vi "DPOAEs_Cecilia_Casarini.vi"() -> ()   [LabVIEW 2015]
uses:
  <vilib>/Utility/error.llb/DialogType.ctl
  <vilib>/DAQmx/write.llb/DAQmx Write (Analog 1D Wfm NChan NSamp).vi
  <vilib>/DAQmx/read.llb/DAQmx Read (Analog Wfm 1Chan NSamp).vi
  <vilib>/addons/_NISVFA/_Baseband FFT/SVPO Power Spectrum (1 Ch DBL Array).vi
  <vilib>/addons/_NISVFA/_Baseband FFT/subVIs/svfa_Convert to One-Sided Power Spectrum.vi
  <vilib>/Analysis/2dsp.llb/Power Spectrum.vi
  <vilib>/Analysis/2dsp.llb/Power Spectrum (DBL).vi
  <vilib>/addons/_NISVFA/_Shared subVIs/Windowing/svfa_Scaled Time Domain Window (Array).vi
  <vilib>/Analysis/4window.llb/Force Window.vi
  <vilib>/Analysis/4window.llb/Force Window (DBL).vi
  <vilib>/Analysis/4window.llb/Exponential Window.vi
  <vilib>/Analysis/4window.llb/Exponential Window (DBL).vi
  <vilib>/DAQmx/create/channels.llb/DAQmx Create Channel (AI-Voltage-Basic).vi
  <vilib>/DAQmx/create/channels.llb/DAQmx Create Channel (AO-Voltage-Basic).vi
  <vilib>/DAQmx/configure/timing.llb/DAQmx Timing (Sample Clock).vi
  <vilib>/DAQmx/configure/trigger.llb/DAQmx Start Trigger (Digital Edge).vi
  <vilib>/DAQmx/miscellaneous.llb/DAQmx Fill In Error Info.vi
  <vilib>/addons/_NISVFA/_Spectrum Processing/subVIs/svfa_Spectrum Info Window to windowTd Type Def.vi
  <vilib>/Analysis/0measdsp.llb/Scaled Time Domain Window.vi
  <vilib>/Analysis/0measdsp.llb/Scaled Time Domain Window (DBL).vi
  <vilib>/Utility/error.llb/Error Cluster From Error Code.vi
panel:
  in  "Frequency of Sine Tone AO-1":dbl=1000.0 format="%0.2p"
  in  "Amplitude of Sine Tone AO-1":dbl=1.0 format="%0.2p"
  out "Non-aligned output/input waveforms":waveform(dbl)(graph)
  in  "Number of extra samples \nto READ from ADC":i32=200
  out "Input spectrum":cluster{"f0":dbl, "df":dbl, "magnitude":dbl[]}(graph)
  out "number of samples \nwritten per channel":u32
  in  "Frequency of Sine Tone AO-0 2":dbl=1000.0 format="%0.2p"
  in  "Amplitude of Sine Tone AO-0":dbl=1.0 format="%0.2p"
  in  "sampling info":cluster{"Fs":dbl, "samples in waveform":dbl}={"Fs"=204800.0, "samples in waveform"=1024.0} {"Fs" format="%.2p"}
  out "buffer size":i32
  in  "minimum value":dbl=-5.0 caption="Output Minimum Value" format="%0.2f"
  in  "maximum value":dbl=5.0 caption="Output Maximum Value" format="%0.2f"
  in  "physical channels":tag="PXI1Slot5/ao0" caption="Output Physical Channels"
  in  "Maximum Value":dbl=5.0 caption="Input Maximum Value" format="%0.2f"
  in  "Minimum Value":dbl=-5.0 caption="Input Minimum Value" format="%0.2f"
  in  "Physical Channel":tag="PXI1Slot5/ai0" caption="Input Physical Channel"
  out "Output waveform (samples)":waveform(dbl)[](graph)
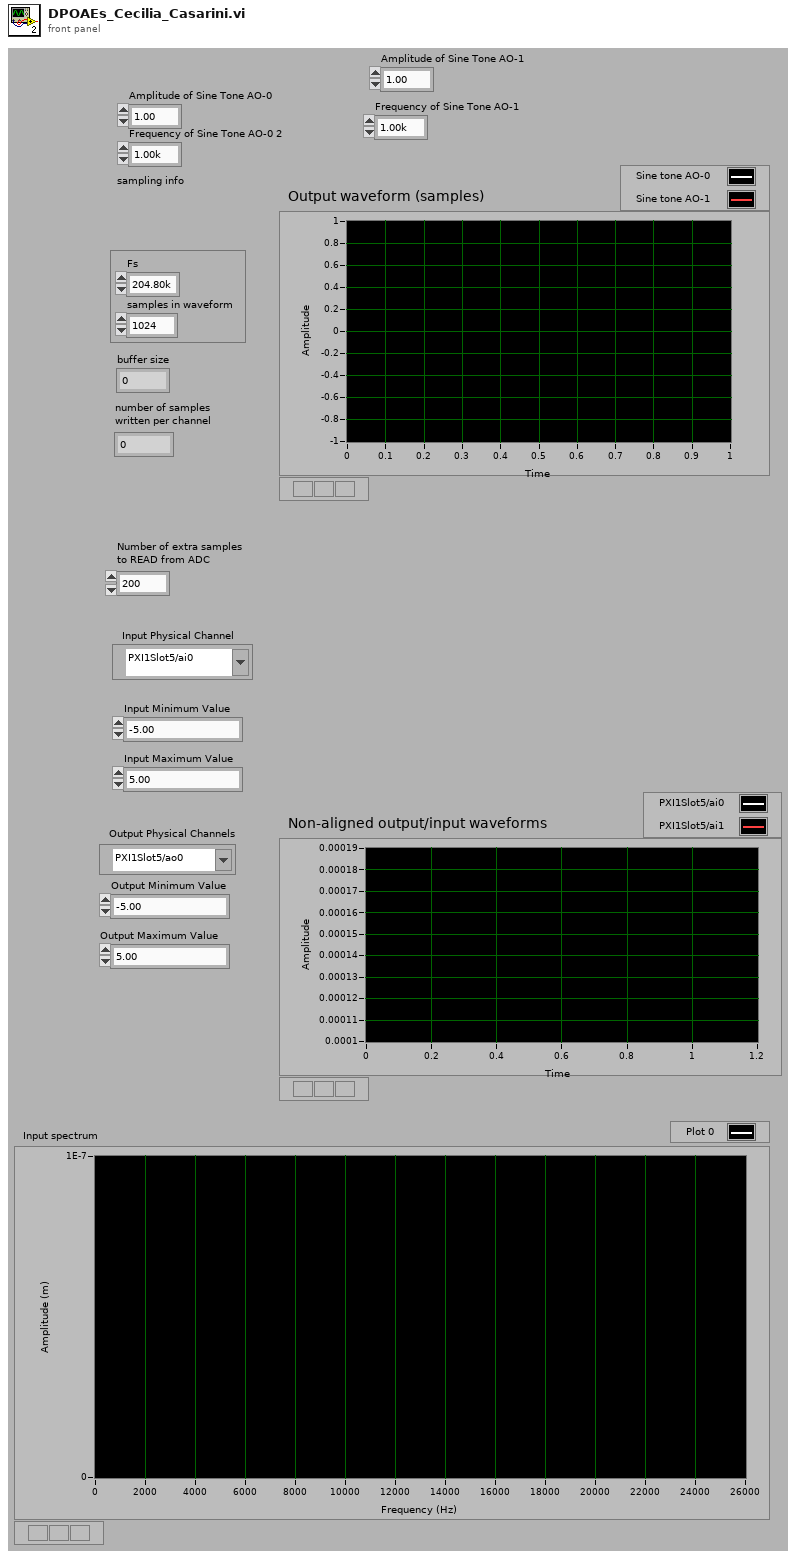
[diagram p1: front panel]
types:
  T1 = typedef "DialogType.ctl" = u16
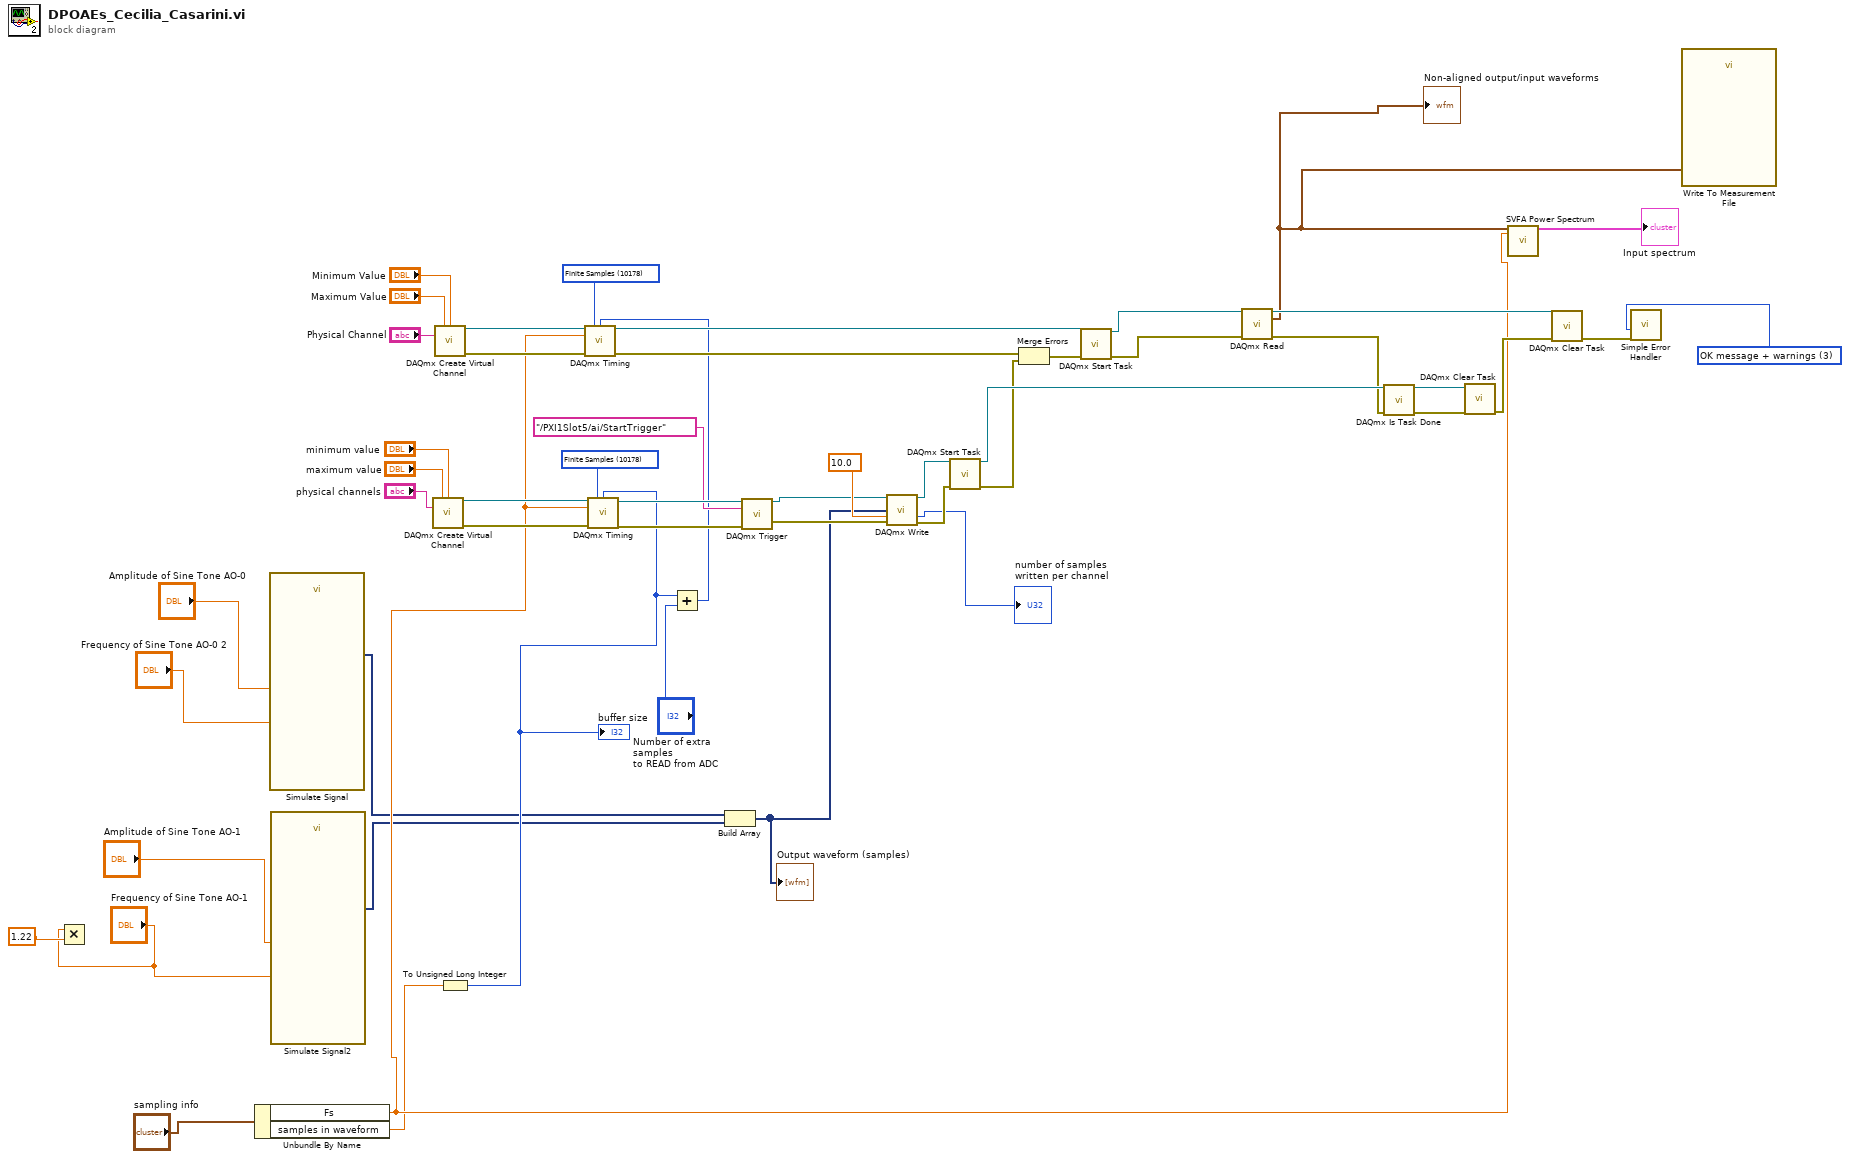
[diagram p0: block diagram]
diagram:
  w24 = T1 3 items=["no dialog", "OK message", "continue or stop message", "OK message + warnings", "continue/stop + warnings"] ("type of dialog (OK msg:1)")
  w44 = 10178 items=["Finite Samples"=10178, "Continuous Samples"=10123] ("sample mode")
  w49 = 10178 items=["Finite Samples"=10178, "Continuous Samples"=10123] ("sample mode")
  n1 = Multiply(x="Frequency of Sine Tone AO-1", y=1.22) -> ()  [unwired: 1 out]
  n2 = Unbundle By Name("sampling info") -> ("Fs"=w13:dbl, "samples in waveform"=w12:dbl)
  n3 = call "Simulate Signal"("Frequency"="Frequency of Sine Tone AO-0 2", "Amplitude"="Amplitude of Sine Tone AO-0") -> ("Sine tone AO-0"=w7:dynamicdata)  [unwired: 12 in, 1 out]
  n4 = call "Simulate Signal2"("Frequency"="Frequency of Sine Tone AO-1", "Amplitude"="Amplitude of Sine Tone AO-1") -> ("Sine tone AO-1"=w6:dynamicdata)  [unwired: 12 in, 1 out]
  n5 = call-poly <vilib>:"DAQmx Create Virtual Channel.vi"("maximum value"="maximum value", "minimum value"="minimum value", "physical channels"="physical channels") -> ("task out"=w43:refnum<k21>, "error out"=w42:errorcluster)  [unwired: 11 in]
  n6 = call-poly <vilib>:"DAQmx Create Virtual Channel.vi"("maximum value"="Maximum Value", "minimum value"="Minimum Value", "physical channels"="Physical Channel") -> ("task out"=w47:refnum<k21>, "error out"=w48:errorcluster)  [unwired: 11 in]
  n7 = To Unsigned Long Integer(number=w12) -> (unsigned 32bit integer=w11:u32)
  "buffer size" <- w11
  n8 = call-poly <vilib>:"DAQmx Timing.vi"("task/channels in"=w43, "sample mode"=w44, "samples per channel"=w11, "rate"=w13, "error in"=w42) -> ("task out"=w37:refnum<k21>, "error out"=w38:errorcluster)  [unwired: 9 in]
  n9 = Add(x=w11, y="Number of extra samples \nto READ from ADC") -> (x+y=w18:u32)
  n10 = call-poly <vilib>:"DAQmx Timing.vi"("task/channels in"=w47, "sample mode"=w49, "samples per channel"=w18, "rate"=w13, "error in"=w48) -> ("task out"=w21:refnum<k21>, "error out"=w22:errorcluster)  [unwired: 9 in]
  n11 = Build Array(w7, w6) -> (w9:dynamicdata[])
  "Output waveform (samples)" <- w9
  n12 = call-poly <vilib>:"DAQmx Trigger.vi"("task/channels in"=w37, "source"=tag "/PXI1Slot5/ai/StartTrigger", "error in"=w38) -> ("task out"=w32:refnum<k21>, "error out"=w33:errorcluster)  [unwired: 11 in]
  n13 = call-poly <vilib>:"DAQmx Write.vi"("task/channels in"=w32, "data"=w9, "timeout"=10.0 ("Wirite Timeout"), "error in"=w33) -> ("task out"=w35:refnum<k21>, "number of samples written per channel"=→"number of samples \nwritten per channel":u32, "error out"=w34:errorcluster)  [unwired: 9 in]
  n14 = call <vilib>:"DAQmx Start Task.vi"("task/channels in"=w35, "error in"=w34) -> ("task out"=w39:refnum<k21>, "error out"=w31:errorcluster)  [unwired: 12 in]
  n15 = Merge Errors(w22, w31) -> (w30:errorcluster)
  n16 = call <vilib>:"DAQmx Start Task.vi"("task/channels in"=w21, "error in"=w30) -> ("task out"=w40:refnum<k21>, "error out"=w41:errorcluster)  [unwired: 12 in]
  n17 = call-poly <vilib>:"DAQmx Read.vi"("task/channels in"=w40, "error in"=w41) -> ("task out"=w26:refnum<k21>, "data"=w1:waveform(dbl), "error out"=w17:errorcluster)  [unwired: 11 in]
  "Non-aligned output/input waveforms" <- w1
  n18 = call <vilib>:"DAQmx Is Task Done.vi"("task/channels in"=w39, "error in"=w17) -> ("task out"=w27:refnum<k21>, "error out"=w25:errorcluster)  [unwired: 11 in, 1 out]
  n19 = call <vilib>:"DAQmx Clear Task.vi"("task in"=w27, "error in"=w25) -> ("error out"=w16:errorcluster)  [unwired: 13 in]
  n20 = call-poly <vilib>:"SVFA Power Spectrum.vi"("scaled signal [EU]"=w1, "sampling rate [Hz]"=w13) -> ("power spectrum [EU^2 rms]"=→"Input spectrum":cluster{"f0":dbl, "df":dbl, "magnitude":dbl[]})  [unwired: 15 in, 2 out]
  n21 = call <vilib>:"DAQmx Clear Task.vi"("task in"=w26, "error in"=w16) -> ("error out"=w15:errorcluster)  [unwired: 13 in]
  n22 = call <vilib>:"Simple Error Handler.vi"("type of dialog (OK msg:1)"=w24, "error in (no error)"=w15) -> ()  [unwired: 3 in, 5 out]
  n23 = call "Write To Measurement File"("Signals"=w1) -> ()  [unwired: 16 in, 3 out]
